vi "RunAllTests.vi"() -> ()   [LabVIEW 2019, in "AssertionTest.lvlib"]
uses:
  AssertionTest.lvlib
  AssertTrue/AssertTrue.lvlib
  AssertFalse/AssertFalse.lvlib
  AssertCount/AssertCount.lvlib
panel:
  out "error out":errorcluster
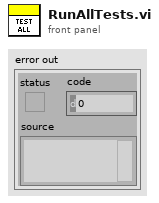
[diagram p1: front panel]
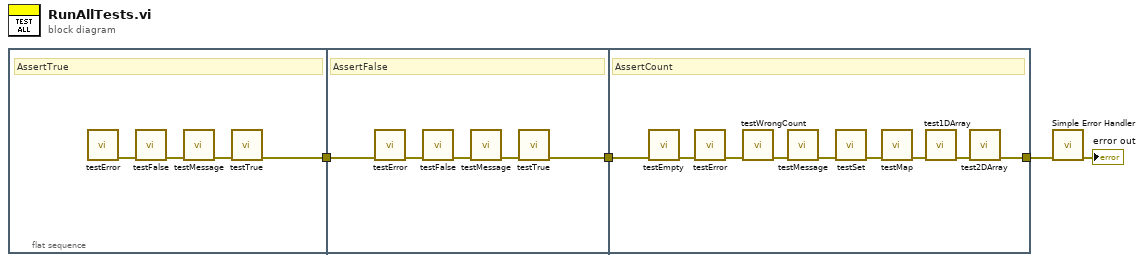
[diagram p0: block diagram]
diagram:
  n1 = flat-sequence {
    tunnel: [w5] -> w4
    tunnel: w4 -> [w13]
    tunnel: [w9] -> w1
    tunnel: [w14] -> w3
    tunnel: w1 -> [w22]
    frame #0 {
      # "AssertTrue"
      n2 = call "testError.vi"() -> ("error out"=w8:errorcluster)  [unwired: 11 in]
      n3 = call "testFalse.vi"("error in (no error)"=w8) -> ("error out"=w7:errorcluster)  [unwired: 10 in]
      n4 = call "testMessage.vi"("error in (no error)"=w7) -> ("error out"=w6:errorcluster)  [unwired: 10 in]
      n5 = call "testTrue.vi"("error in (no error)"=w6) -> ("error out"=w5:errorcluster)  [unwired: 10 in]
    }
    frame #1 {
      # "AssertFalse"
      n6 = call "testError.vi"("error in (no error)"=w13) -> ("error out"=w12:errorcluster)  [unwired: 10 in]
      n7 = call "testFalse.vi"("error in (no error)"=w12) -> ("error out"=w11:errorcluster)  [unwired: 10 in]
      n8 = call "testMessage.vi"("error in (no error)"=w11) -> ("error out"=w10:errorcluster)  [unwired: 10 in]
      n9 = call "testTrue.vi"("error in (no error)"=w10) -> ("error out"=w9:errorcluster)  [unwired: 10 in]
    }
    frame #2 {
      # "AssertCount"
      n10 = call "testEmpty.vi"("error in (no error)"=w22) -> ("error out"=w21:errorcluster)  [unwired: 10 in]
      n11 = call "testError.vi"("error in (no error)"=w21) -> ("error out"=w20:errorcluster)  [unwired: 10 in]
      n12 = call "testWrongCount.vi"("error in (no error)"=w20) -> ("error out"=w19:errorcluster)  [unwired: 10 in]
      n13 = call "testMessage.vi"("error in (no error)"=w19) -> ("error out"=w18:errorcluster)  [unwired: 10 in]
      n14 = call "testSet.vi"("error in (no error)"=w18) -> ("error out"=w17:errorcluster)  [unwired: 10 in]
      n15 = call "testMap.vi"("error in (no error)"=w17) -> ("error out"=w16:errorcluster)  [unwired: 10 in]
      n16 = call "test1DArray.vi"("error in (no error)"=w16) -> ("error out"=w15:errorcluster)  [unwired: 10 in]
      n17 = call "test2DArray.vi"("error in (no error)"=w15) -> ("error out"=w14:errorcluster)  [unwired: 10 in]
    }
  }
  n18 = call <vilib>:"Simple Error Handler.vi"("error in (no error)"=w3) -> ("error out"=→"error out":errorcluster)  [unwired: 4 in, 4 out]
